vi "Sum in Tiles.vi"(10 "size":i32, 11 "Image":i64[][](array[numeric])) -> (1 "Max Index":i32[](array[numeric]), 2 "Maximum":i64, 3 "Counts in Tiles":i64[][](array[numeric]))   [LabVIEW 2014]
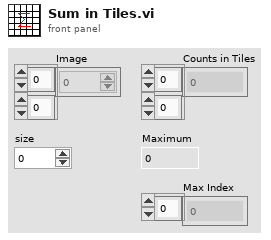
[diagram p1: front panel]
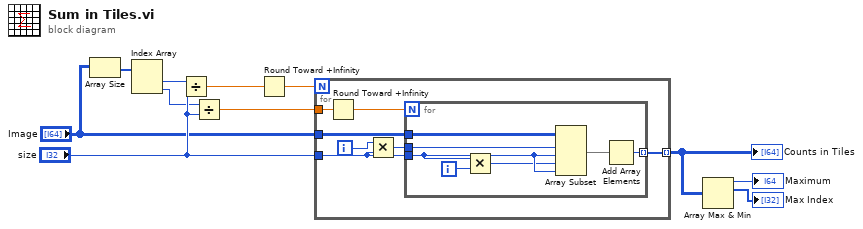
[diagram p0: block diagram]
diagram:
  n1 = Array Size(array="Image") -> (size(s)=w2:i32[])
  n2 = Index Array(array=w2) -> (element #1=w3:i32, element #2=w4:i32)  [unwired: 2 in]
  n3 = Divide(x=w3, y="size") -> (x/y=w10:dbl)
  n4 = Divide(x=w4, y="size") -> (x/y=w6:dbl)
  n5 = Round Toward +Infinity(x=w10) -> (ceil(x): smallest int >= x=w11:dbl)
  n6 = for {
    N: w11 -> [_]
    tunnel: "Image" -> [w18]
    tunnel: "size" -> [w16]
    tunnel: w6 -> [w13]
    tunnel: [w14] -> w7 mode=indexing
    i -> [w17]
    n7 = Round Toward +Infinity(x=w13) -> (ceil(x): smallest int >= x=w12:dbl)
    n8 = Multiply(x=w17, y=w16) -> (x*y=w15:i32)
    n9 = for {
      N: w12 -> [_]
      tunnel: w18 -> [w25]
      tunnel: w15 -> [w24]
      tunnel: w16 -> [w22]
      tunnel: [w20] -> w14 mode=indexing
      i -> [w23]
      n10 = Multiply(x=w22, y=w23) -> (x*y=w21:i32)
      n11 = Array Subset(array=w25, index (row)=w24, length (row)=w22, index (col)=w21, length (col)=w22) -> (w19:i64[][])
      n12 = Add Array Elements(numeric array=w19) -> (sum=w20:i64)
    }
  }
  "Counts in Tiles" <- w7
  n13 = Array Max & Min(array=w7) -> (max value=→"Maximum":i64, max index (indices)=→"Max Index":i32[])  [unwired: 2 out]
